vi "Get All Net Use Mapped Drives.vi"(11 "error in (no error)":errorcluster) -> (4 "Mapped Drive Letters":string[](array[string]), 6 "Mapped Paths":string[](array[string]), 15 "error out":errorcluster)   [LabVIEW 2017, in "G3_Build Process File Utilities.lvlib"]
doc: "Returns an array of all mapped drive letters and a parallel array of all mapped paths."
uses:
  G3_Build Process File Utilities.lvlib
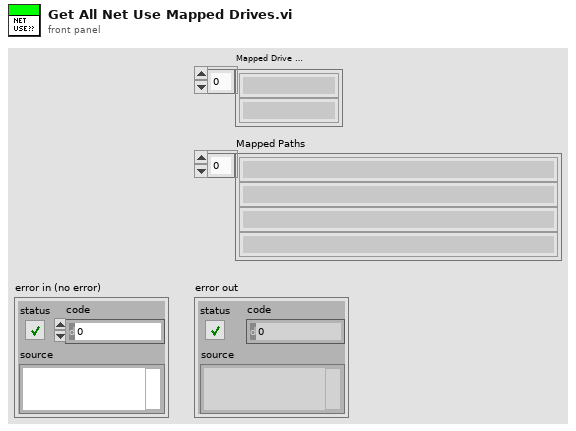
[diagram p1: front panel]
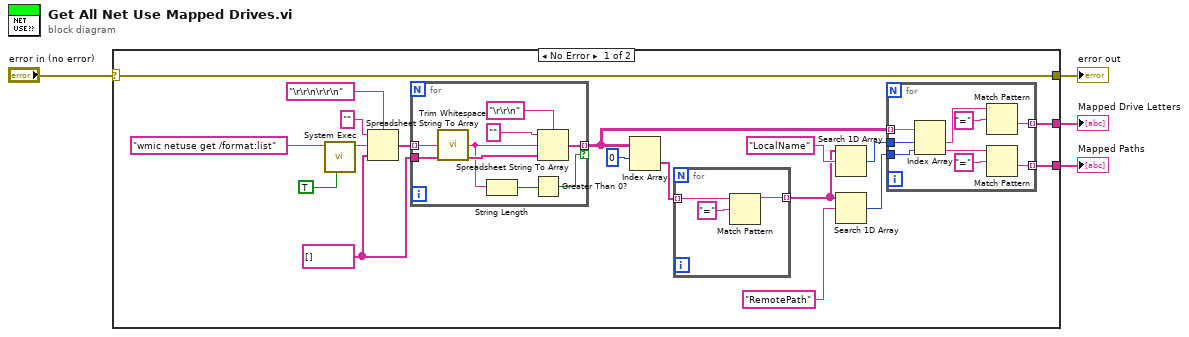
[diagram p0: block diagram]
diagram:
  n1 = case shown="No Error" "error in (no error)" {
    selector: "error in (no error)" -> [w5 w43]
    tunnel: [w7 _] -> w4
    tunnel: [w6 _] -> w3
    tunnel: [w5 w43] -> w1
    frame No Error {
      w16 = string[] []
      n2 = call <vilib>:"System Exec.vi"("run minimized? (F)"=TRUE, "command line"="wmic netuse get /format:list") -> ("standard output"=w20:string)  [unwired: 6 in, 3 out]
      n3 = Spreadsheet String To Array(delimiter (Tab)="\r\r\n\r\r\n", format string="", spreadsheet string=w20, array type (2D Dbl)=w16) -> (array=w17:string[])
      n4 = for {
        tunnel: w17 -> [w42] mode=indexing
        tunnel: w16 -> [w40]
        tunnel: [w37] -> w10 mode=indexing if=w36
        n5 = call <vilib>:"Trim Whitespace.vi"("string"=w42) -> ("trimmed string"=w39:string)  [unwired: 1 in]
        n6 = String Length(string=w39) -> (length=w41:i32)
        n7 = Greater Than 0?(x=w41) -> (x > 0?=w36:bool)
        n8 = Spreadsheet String To Array(delimiter (Tab)="\r\r\n", format string="", spreadsheet string=w39, array type (2D Dbl)=w40) -> (array=w37:string[])
      }
      n9 = Index Array(array=w10, index (row)=0) -> (element=w14:string[])  [unwired: 1 in]
      n10 = for {
        tunnel: w14 -> [w34] mode=indexing
        tunnel: [w32] -> w12 mode=indexing
        n11 = Match Pattern(string=w34, regular expression="=") -> (before substring=w32:string)  [unwired: 1 in, 3 out]
      }
      n12 = Search 1D Array(1D array=w12, element="LocalName") -> (index of element=w9:i32)  [unwired: 1 in]
      n13 = Search 1D Array(1D array=w12, element="RemotePath") -> (index of element=w8:i32)  [unwired: 1 in]
      n14 = for {
        tunnel: w10 -> [w31] mode=indexing
        tunnel: w9 -> [w30]
        tunnel: w8 -> [w29]
        tunnel: [w24] -> w7 mode=indexing
        tunnel: [w23] -> w6 mode=indexing
        n15 = Index Array(array=w31, index #1=w30, index #2=w29) -> (element #1=w27:string, element #2=w26:string)
        n16 = Match Pattern(string=w27, regular expression="=") -> (after substring=w24:string)  [unwired: 1 in, 3 out]
        n17 = Match Pattern(string=w26, regular expression="=") -> (after substring=w23:string)  [unwired: 1 in, 3 out]
      }
    }
    frame Error {
    }
  }
  "Mapped Drive Letters" <- w4
  "Mapped Paths" <- w3
  "error out" <- w1
